vi "Inverse f Filter Coefficients.vi"(8 "unity gain freq (rad/s)":dbl=1.0 format="%.2g", 9 "filter specifications":T4={"lower cutoff freq"=0.1, "higher cutoff freq"=100.0, "order"=5}, 10 "fs":dbl=1000.0 format="%.2f", 11 "exponent":dbl=1.0 format="%.2g") -> (0 "error":i32, 1 "magnitude error (dB)":T1, 2 "filter information":T2, 3 "IIR Filter Cluster":T3 {"Forward Coefficients" format="%.4f"; "Reverse Coefficients" format="%.4f"}, 4 "noise bandwidth":dbl=1.0 format="%.2g")   [LabVIEW 2020, in "NI_AALBase.lvlib"]
doc: "Designs an IIR filter whose magnitude-squared response is inversely proportional to frequency over a specified frequency range. This inverse-f filter is typically used to colorize spectrally flat, or white, noise."
uses:
  NI_AALBase.lvlib
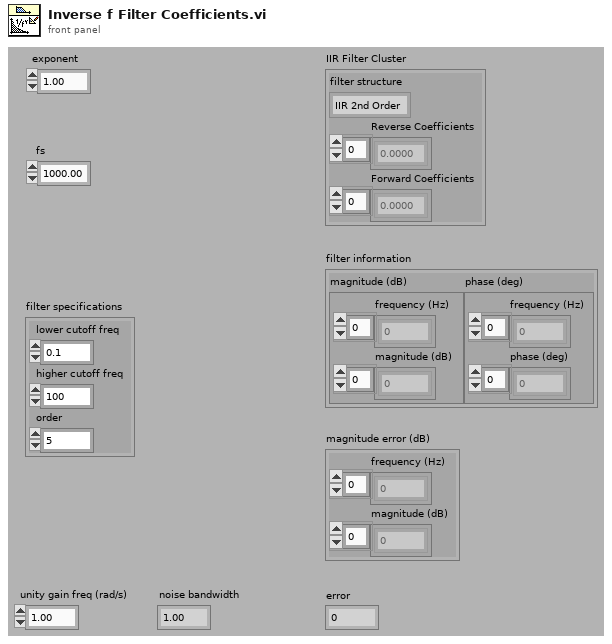
[diagram p1: front panel]
types:
  T1 = cluster{"frequency (Hz)":dbl[], "magnitude (dB)":dbl[]}
  T2 = cluster{"magnitude (dB)":cluster{"frequency (Hz)":dbl[], "magnitude (dB)":dbl[]}, "phase (deg)":cluster{"frequency (Hz)":dbl[], "phase (deg)":dbl[]}}
  T3 = cluster{"filter structure":enum32{"IIR 2nd Order", "IIR 4th Order"}, "Reverse Coefficients":dbl[], "Forward Coefficients":dbl[]}
  T4 = cluster{"lower cutoff freq":dbl, "higher cutoff freq":dbl, "order":i32}
  T5 = cluster{"Fstart":dbl, "Fstop":dbl, "# points":i32, "type":u16}
  T6 = cluster{"filter structure":enum32{"IIR 2nd Order", "IIR 4th Order"}, "b[i]":dbl[], "b[i]":dbl[]}
  T7 = cluster{"corrected magnitude (dB)":cluster{"frequency (Hz)":dbl[], "magnitude (dB)":dbl[]}, "Phase (degrees)":cluster{dbl[], dbl[]}}
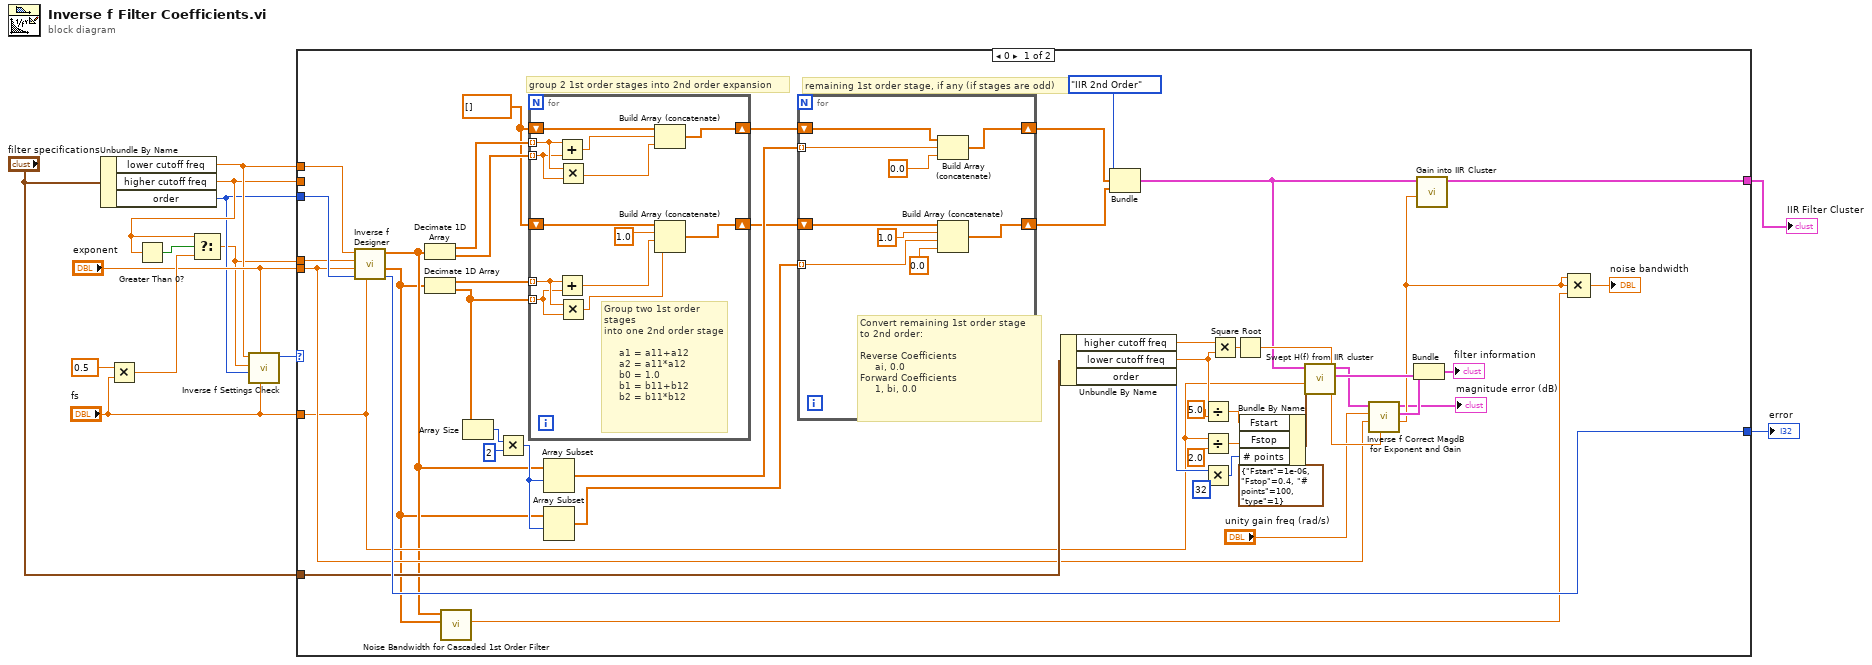
[diagram p0: block diagram]
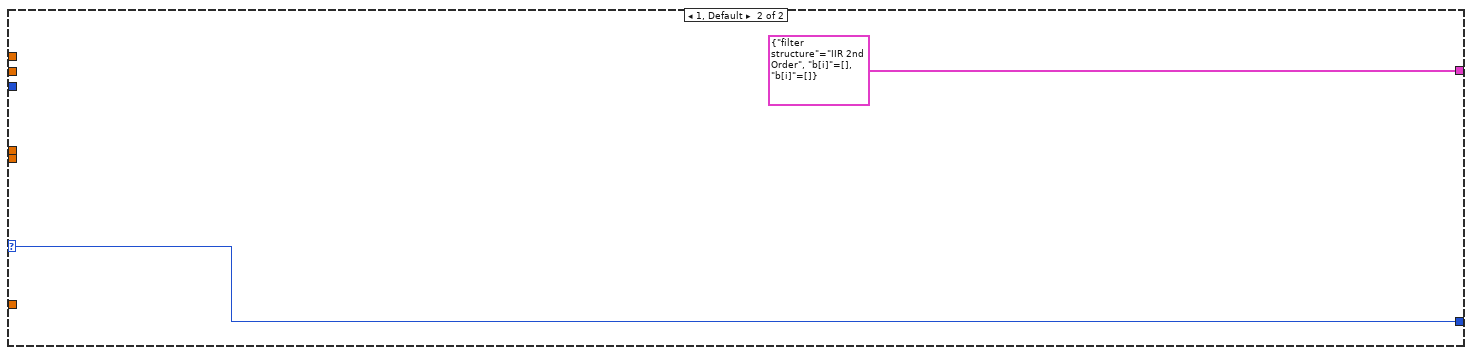
[diagram p2: hidden frame]
diagram:
  n1 = Unbundle By Name("filter specifications") -> ("lower cutoff freq"=w7:dbl, "higher cutoff freq"=w6:dbl, "order"=w5:i32)
  n2 = Multiply(x=0.5 ("y"), y="fs") -> (x*y=w11:dbl)
  n3 = Greater Than 0?(x=w6) -> (x > 0?=w13:bool)
  n4 = Select(t=w6, s=w13, f=w11) -> (s? t:f=w4:dbl)
  n5 = call "Inverse f Settings Check.vi"("fs"="fs", "exponent"="exponent", "order"=w5, "higher cutoff freq"=w4, "lower cutoff freq"=w7) -> ("error code"=w3:i32)  [unwired: 5 in, 1 out]
  n6 = case shown="0" w3 {
    selector: w3 -> [_ w84]
    tunnel: "exponent" -> [w24 _]
    tunnel: [w21 T6 {"filter structure"=enum."IIR 2nd Order", "b[i]"=[], "b[i]"=[]}] -> w1
    tunnel: "fs" -> [w23 _]
    tunnel: w4 -> [w43 _]
    tunnel: [w46 w84] -> w9
    tunnel: w7 -> [w45 _]
    tunnel: w6 -> [_ _]
    tunnel: w5 -> [w44 _]
    tunnel: "filter specifications" -> [w26 _]
    frame 0 {
      w48 = dbl[] [] ("b[i]")
      # "group 2 1st order stages into 2nd order expansion"
      # "remaining 1st order stage, if any (if stages are odd)"
      n7 = call "Inverse f Designer.vi"("fs"=w23, "order"=w44, "exponent"=w24, "higher cutoff freq"=w43, "lower cutoff freq"=w45) -> ("error"=w46:i32, "b[i]"=w19:dbl[], "a[i]"=w20:dbl[])  [unwired: 1 in, 1 out]
      n8 = Decimate 1D Array(w20) -> (w52:dbl[], w51:dbl[])
      n9 = Decimate 1D Array(w19) -> (w50:dbl[], w49:dbl[])
      n10 = call "Noise Bandwidth for Cascaded 1st Order Filter.vi"("b[i]"=w19, "a[i]"=w20) -> ("noise bandwidth"=w18:dbl)  [unwired: 9 in]
      n11 = Array Size(array=w49) -> (size(s)=w58:i32)
      n12 = Multiply(x=w58, y=2) -> (x*y=w56:i32)
      n13 = for {
        shift-right: [w72] -> w47
        shift-left: w48 -> [w73]
        shift-right: [w71] -> w53
        shift-left: w48 -> [w74]
        tunnel: w52 -> [w68] mode=indexing
        tunnel: w51 -> [w67] mode=indexing
        tunnel: w50 -> [w66] mode=indexing
        tunnel: w49 -> [w65] mode=indexing
        # "Group two 1st order stages\ninto one 2nd order stage\n\n     a1 = a11+a12\n     a2 = a11*a12\n     b0 = 1.0\n     b1 = b11+b12\n     b2 = b11*b12"
        n14 = Add(x=w68, y=w67) -> (x+y=w69:dbl)
        n15 = Add(x=w66, y=w65) -> (x+y=w64:dbl)
        n16 = Multiply(x=w68, y=w67) -> (x*y=w63:dbl)
        n17 = Multiply(x=w66, y=w65) -> (x*y=w62:dbl)
        n18 = Build Array (concatenate)(w73, w69, w63) -> (w72:dbl[])
        n19 = Build Array (concatenate)(w74, 1.0, w64, w62) -> (w71:dbl[])
      }
      n20 = Array Subset(array=w20, index=w56) -> (w55:dbl[])  [unwired: 1 in]
      n21 = Array Subset(array=w19, index=w56) -> (w54:dbl[])  [unwired: 1 in]
      n22 = for {
        shift-right: [w81] -> w61
        shift-left: w47 -> [w82]
        shift-right: [w80] -> w60
        shift-left: w53 -> [w83]
        tunnel: w55 -> [w76] mode=indexing
        tunnel: w54 -> [w75] mode=indexing
        # "Convert remaining 1st order stage \nto 2nd order:\n\nReverse Coefficients\n     ai, 0.0\nForward Coefficients\n     1, bi, 0.0"
        n23 = Build Array (concatenate)(w82, w76, 0.0) -> (w81:dbl[])
        n24 = Build Array (concatenate)(w83, 1.0, w75, 0.0) -> (w80:dbl[])
      }
      n25 = Unbundle By Name(w26) -> ("higher cutoff freq"=w31:dbl, "lower cutoff freq"=w30:dbl, "order"=w36:i32)
      n26 = Bundle("filter structure"=enum32{"IIR 2nd Order", "IIR 4th Order"}."IIR 2nd Order", "b[i]"=w61, "b[i]"=w60) -> (w22:T6)  [unwired: 1 in]
      n27 = Divide(x=w30, y=5.0) -> (x/y=w33:dbl)
      n28 = Divide(x=w23, y=2.0) -> (x/y=w32:dbl)
      n29 = Multiply(x=w36, y=32) -> (x*y=w37:i32)
      n30 = Multiply(x=w31, y=w30) -> (x*y=w29:dbl)
      n31 = Square Root(x=w29) -> (sqrt(x)=w28:dbl)
      n32 = Bundle By Name(cluster=T5 {"Fstart"=1e-06, "Fstop"=0.4, "# points"=100, "type"=1} ("Sweep specs"), "Fstart"=w33, "Fstop"=w32, "# points"=w37) -> (w34:T5)
      n33 = call "Swept H(f) from IIR cluster.vi"("Sweep specs"=w34, "Fs"=w23, "IIR Filter Cluster"=w22) -> ("Phase (degrees)"=w40:cluster{dbl[], dbl[]}, "Magnitude (dB)"=w35:cluster{dbl[], dbl[]})  [unwired: 7 in]
      n34 = call "Inverse f Correct MagdB for Exponent and Gain.vi"("alignment frequency (Hz)"=w28, "exponent"=w24, "unity gain freq (rd/s)"="unity gain freq (rad/s)", "magnitude (dB)"=w35) -> ("gain to apply"=w17:dbl, "corrected magnitude (dB)"=w27:T1, "magnitude error (dB)"=→"magnitude error (dB)":T1)  [unwired: 5 in]
      n35 = Bundle("corrected magnitude (dB)"=w27, "Phase (degrees)"=w40) -> (→"filter information":T7)  [unwired: 1 in]
      n36 = call "Gain into IIR Cluster.vi"("gain"=w17, "IIR Filter Cluster in"=w22) -> ("IIR Filter Cluster out"=w21:T3)  [unwired: 9 in]
      n37 = Compound Arithmetic op=MULTIPLY(w17, w17, w18) -> (→"noise bandwidth":dbl)
    }
    frame 1, Default {
    }
  }
  "error" <- w9
  "IIR Filter Cluster" <- w1
